vi "To Variant.vi"(8 "error in":errorcluster, 11 "Data Type in":refnum<class "Data Type.lvclass">) -> (0 "error out":errorcluster, 3 "Variant":variant)   [LabVIEW 2017, in "Data Type.lvclass"]
uses:
  <vilib>/gpm_packages/@cs/data-type-serializer/source/Data Type/Data Type.lvclass
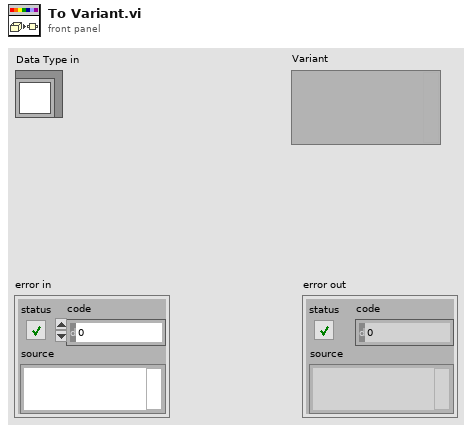
[diagram p1: front panel]
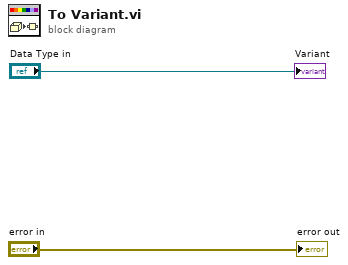
[diagram p0: block diagram]
diagram:
  "Variant" <- "Data Type in"
  "error out" <- "error in"
